vi "TCP Send Percent.vi"(8 "error in":errorcluster, 11 "Percent":dbl=50.0) -> (0 "error out":errorcluster)   [LabVIEW 2013]
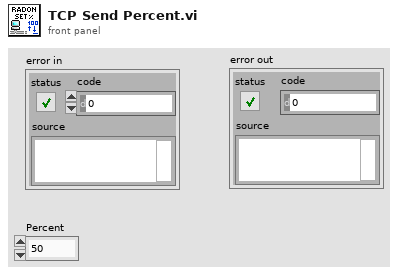
[diagram p1: front panel]
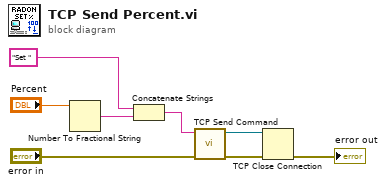
[diagram p0: block diagram]
diagram:
  n1 = Number To Fractional String(number="Percent") -> (F-format string=w6:string)  [unwired: 3 in]
  n2 = Concatenate Strings("Set " ("Command"), w6) -> (w4:string)
  n3 = call "TCP Send Command.vi"("error in"="error in", "Command"=w4) -> ("error out"=w3:errorcluster, "connection ID out"=w1:refnum<k5>)  [unwired: 8 in]
  n4 = TCP Close Connection(connection ID=w1, error in (no error)=w3) -> (error out=→"error out":errorcluster)  [unwired: 1 in, 1 out]
